vi "niWLAN - 80211abgnIQMeasurementsSettings_5663.vi"(0 "niwlan analysis session":T6, 1 "WLAN Measurement Settings":T1={"OFDM Advanced Controls(11ag)"={"OFDM Auto Compute Acquisition Length Enabled"=0, "OFDM Maximum Symbols Used"=0, "OFDM Time Tracking Enabled"=0, "OFDM Channel Tracking Enabled"=0, "OFDM Amplitude Tracking Enabled"=1, "OFDM CFO Estimation Method"=0, "OFDM Phase Tracking Method"=0, "OFDM Header Detection Enabled"=0, "OFDM MAC FCS Check Enabled"=0, "#Avg"=10, "#Iterations"=10}, "DSSS Demod Parameters"={"DSSS Auto Compute Acquisition Length Enabled"=0, "DSSS Equalization Enabled"=0, "DSSS Header Detection Enabled"=0, "DSSS MAC FCS Check Enabled"=0, "DSSS Measurement Start Location"=0, "DSSS Phase Tracking Method"=0, "DSSS Maximum Chips Used"=0, "DSSS Reference Pulse Shaping Filter"=0, "DSSS Reference Pulse Shaping Filter Coefficient"=0.0, "# Avg"=1024, "# Iterations"=1024, "DSSS Power Ramp Enabled"=0}, "OFDM Advanced Controls (11n)"={"OFDM Auto Compute Acquisition Length Enabled"=0, "OFDM Maximum Symbols Used"=0, "OFDM Time Tracking Enabled"=0, "OFDM Channel Tracking Enabled"=0, "OFDM Amplitude Tracking Enabled"=1, "OFDM CFO Estimation Method"=0, "OFDM Phase Tracking Method"=0, "OFDM Header Detection Enabled"=0, "OFDM MAC FCS Check Enabled"=0, "#Avg"=10, "#Iterations"=10}, "OFDM Advanced Controls(11ac)"={"OFDM Auto Compute Acquisition Length Enabled"=0, "OFDM Maximum Symbols Used"=0, "OFDM Time Tracking Enabled"=1, "OFDM Channel Tracking Enabled"=0, "OFDM Amplitude Tracking Enabled"=0, "OFDM CFO Estimation Method"=0, "OFDM Phase Tracking Method"=0, "OFDM Header Detection Enabled"=0, "OFDM MAC FCS Check Enabled"=0, "#Avg"=10, "#Iterations"=10}} {"OFDM Advanced Controls(11ac)"."OFDM Phase Tracking Method" items=["Standard", "Instantaneous", "None", "Standard with Cubic Spline Fit"]; "OFDM Advanced Controls(11ac)"."OFDM CFO Estimation Method" items=["Preamble Only", "Preamble and Data"]; "OFDM Advanced Controls(11ac)"."OFDM Channel Tracking Enabled" items=["False", "True"]; "OFDM Advanced Controls(11ac)"."OFDM Amplitude Tracking Enabled" items=["False", "True"]; "OFDM Advanced Controls(11ac)"."OFDM Time Tracking Enabled" items=["True"=1, "False"=0]; "OFDM Advanced Controls(11ac)"."OFDM Auto Compute Acquisition Length Enabled" items=["False", "True"]; "OFDM Advanced Controls(11ac)"."OFDM MAC FCS Check Enabled" items=["False", "True"]; "OFDM Advanced Controls(11ac)"."OFDM Header Detection Enabled" items=["False", "True"]; "OFDM Advanced Controls (11n)"."OFDM Phase Tracking Method" items=["Standard", "Instantaneous", "None", "Standard with Cubic Spline Fit"]; "OFDM Advanced Controls (11n)"."OFDM CFO Estimation Method" items=["Preamble Only", "Preamble and Data"]; "OFDM Advanced Controls (11n)"."OFDM Channel Tracking Enabled" items=["False", "True"]; "OFDM Advanced Controls (11n)"."OFDM Amplitude Tracking Enabled" items=["False", "True"]; "OFDM Advanced Controls (11n)"."OFDM Time Tracking Enabled" items=["True"=1, "False"=0]; "OFDM Advanced Controls (11n)"."OFDM Auto Compute Acquisition Length Enabled" items=["False", "True"]; "OFDM Advanced Controls (11n)"."OFDM MAC FCS Check Enabled" items=["False", "True"]; "OFDM Advanced Controls (11n)"."OFDM Header Detection Enabled" items=["False", "True"]; "DSSS Demod Parameters"."DSSS Power Ramp Enabled" items=["False", "True"]; "DSSS Demod Parameters"."DSSS Auto Compute Acquisition Length Enabled" items=["False", "True"]; "DSSS Demod Parameters"."DSSS Phase Tracking Method" items=["Standard", "Instantaneous"]; "DSSS Demod Parameters"."DSSS Equalization Enabled" items=["False", "True"]; "DSSS Demod Parameters"."DSSS Reference Pulse Shaping Filter" items=["Rectangular", "Raised Cosine", "Root Raised Cosine", "Gaussian"]; "DSSS Demod Parameters"."DSSS MAC FCS Check Enabled" items=["False", "True"]; "DSSS Demod Parameters"."DSSS Header Detection Enabled" items=["False", "True"]; "OFDM Advanced Controls(11ag)"."OFDM Phase Tracking Method" items=["Standard", "Instantaneous", "None", "Standard with Cubic Spline Fit"]; "OFDM Advanced Controls(11ag)"."OFDM CFO Estimation Method" items=["Preamble Only", "Preamble and Data"]; "OFDM Advanced Controls(11ag)"."OFDM Channel Tracking Enabled" items=["False", "True"]; "OFDM Advanced Controls(11ag)"."OFDM Amplitude Tracking Enabled" items=["False", "True"]; "OFDM Advanced Controls(11ag)"."OFDM Time Tracking Enabled" items=["True"=1, "False"=0]; "OFDM Advanced Controls(11ag)"."OFDM Auto Compute Acquisition Length Enabled" items=["False", "True"]; "OFDM Advanced Controls(11ag)"."OFDM MAC FCS Check Enabled" items=["False", "True"]; "OFDM Advanced Controls(11ag)"."OFDM Header Detection Enabled" items=["False", "True"]}, 2 "Measurement Type":T4(ring), 5 "TV Parameters(DataType)":T5 {"Standard" items=["80211A/G/J/P OFDM", "80211B/G DSSS", "80211G DSSSOFDM", "80211N MIMOOFDM", "80211AC MIMOOFDM"]; "OFDM Data Rate (Mbps)" items=["6", "9", "12", "18", "24", "36", "48", "54"]; "80211n PLCP Frame Format" items=["Mixed Format", "Greenfield Format"]; "FEC Coding Type" items=["BCC", "LDPC"]; "DSSS Data Rate (Mbps)" items=["1", "2", "5.5 CCK", "5.5 PBCC", "11 CCK", "11 PBCC", "22", "33"]}, 7 "Set TV ?":bool, 11 "error in":errorcluster, 13 "Cal Routine ?":bool) -> (4 "niWLAN session":T6, 15 "error out":errorcluster)   [LabVIEW 2011]
uses:
  <vilib>/RF Toolkits/WLAN/analysis/controls/wlanv1 Analysis Refnum.ctl
  TV/RW/Includes/WLAN - TV - RW - INC - TV_DataType_Cluster.ctl
  TV/RW/Includes/WLAN - TV - RW - INC - Tx_Measurement_Cluster.ctl
  TV/RW/Includes/WLAN - TV - RW - INC - TV_OFDM Demod.ctl
  TV/RW/Includes/WLAN - TV - RW - INC - TV_DSSS Demod.ctl
  Program Files/National Instruments/LabVIEW 2011/resource/objmgr/niWLANAnalysis.rc
panel:
  out "Standard":i32(ring) items=["80211A/G/J/P OFDM", "80211B/G DSSS", "80211G DSSSOFDM", "80211N MIMOOFDM", "80211AC MIMOOFDM"]
  # "Hardware Configuration"
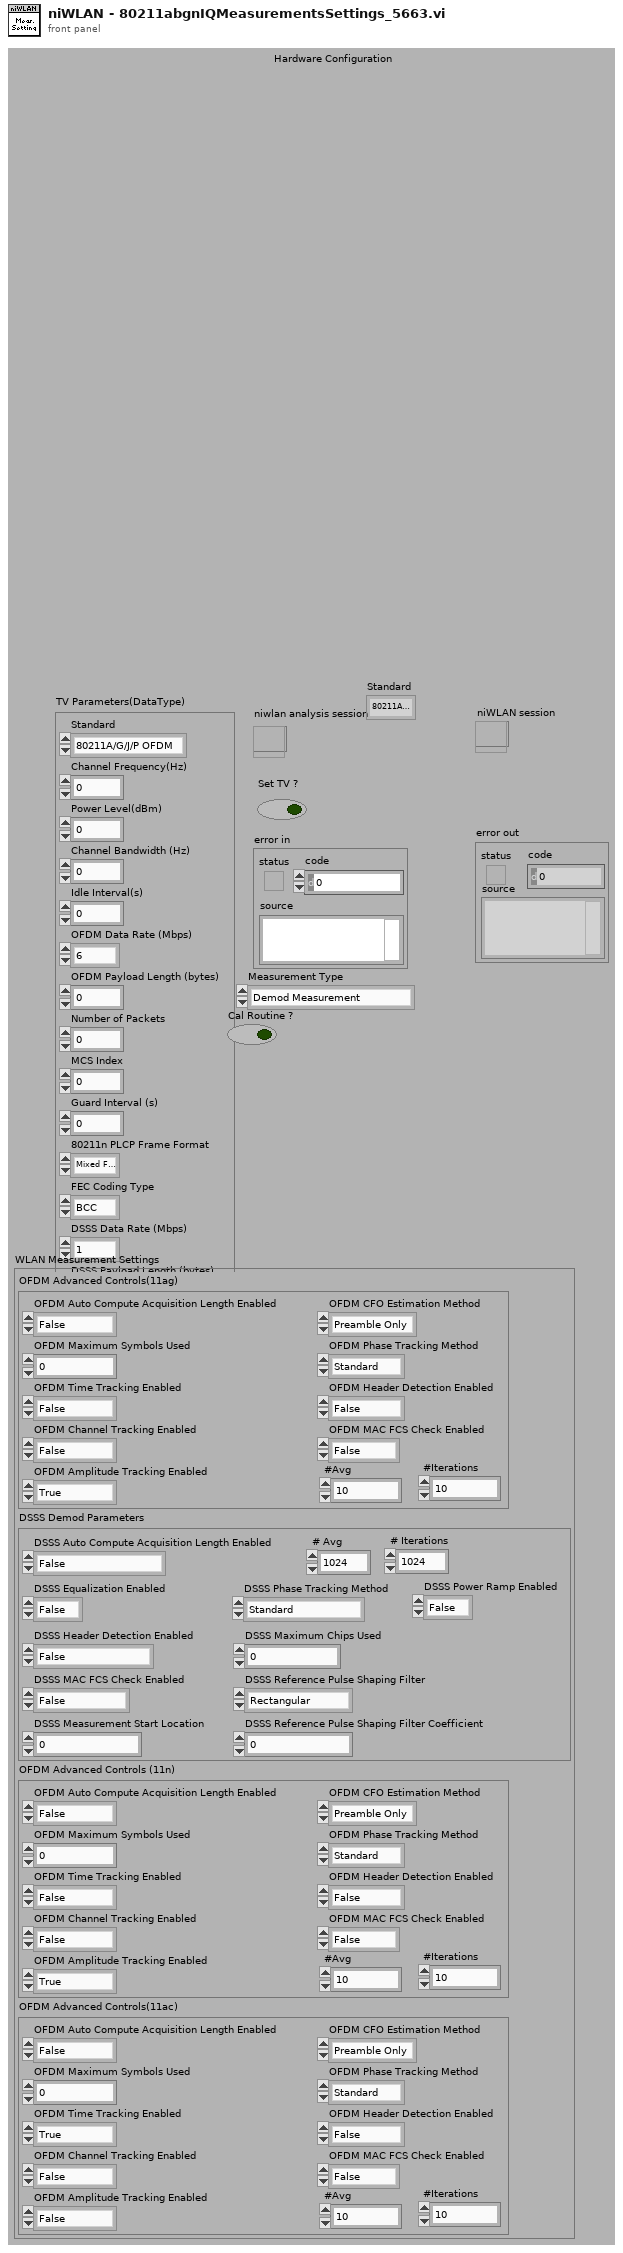
[diagram p1: front panel]
types:
  T1 = typedef "WLAN - TV - RW - INC - Tx_Measurement_Cluster.ctl" = cluster{"OFDM Advanced Controls(11ag)":T2, "DSSS Demod Parameters":T3, "OFDM Advanced Controls (11n)":T2, "OFDM Advanced Controls(11ac)":cluster{"OFDM Auto Compute Acquisition Length Enabled":i32, "OFDM Maximum Symbols Used":i32, "OFDM Time Tracking Enabled":i32, "OFDM Channel Tracking Enabled":i32, "OFDM Amplitude Tracking Enabled":i32, "OFDM CFO Estimation Method":i32, "OFDM Phase Tracking Method":i32, "OFDM Header Detection Enabled":i32, "OFDM MAC FCS Check Enabled":i32, "#Avg":i32, "#Iterations":i32}}
  T2 = typedef "WLAN - TV - RW - INC - TV_OFDM Demod.ctl" = cluster{"OFDM Auto Compute Acquisition Length Enabled":i32, "OFDM Maximum Symbols Used":i32, "OFDM Time Tracking Enabled":i32, "OFDM Channel Tracking Enabled":i32, "OFDM Amplitude Tracking Enabled":i32, "OFDM CFO Estimation Method":i32, "OFDM Phase Tracking Method":i32, "OFDM Header Detection Enabled":i32, "OFDM MAC FCS Check Enabled":i32, "#Avg":i32, "#Iterations":i32}
  T3 = typedef "WLAN - TV - RW - INC - TV_DSSS Demod.ctl" = cluster{"DSSS Auto Compute Acquisition Length Enabled":i32, "DSSS Equalization Enabled":i32, "DSSS Header Detection Enabled":i32, "DSSS MAC FCS Check Enabled":i32, "DSSS Measurement Start Location":i32, "DSSS Phase Tracking Method":i32, "DSSS Maximum Chips Used":i32, "DSSS Reference Pulse Shaping Filter":i32, "DSSS Reference Pulse Shaping Filter Coefficient":dbl, "# Avg":i32, "# Iterations":i32, "DSSS Power Ramp Enabled":i32}
  T4 = enum16{"Demod Measurement", "Spectrum Measurement"}
  T5 = typedef "WLAN - TV - RW - INC - TV_DataType_Cluster.ctl" = cluster{"Standard":i32, "Channel Frequency(Hz)":dbl, "Power Level(dBm)":dbl, "Channel Bandwidth (Hz)":dbl, "Idle Interval(s)":dbl, "OFDM Data Rate (Mbps)":i32, "OFDM Payload Length (bytes)":i32, "Number of Packets":i32, "MCS Index":i32, "Guard Interval (s)":dbl, "80211n PLCP Frame Format":i32, "FEC Coding Type":i32, "DSSS Data Rate (Mbps)":i32, "DSSS Payload Length (bytes)":i32, "N_SS":i32}
  T6 = typedef "wlanv1 Analysis Refnum.ctl" = refnum<k20>
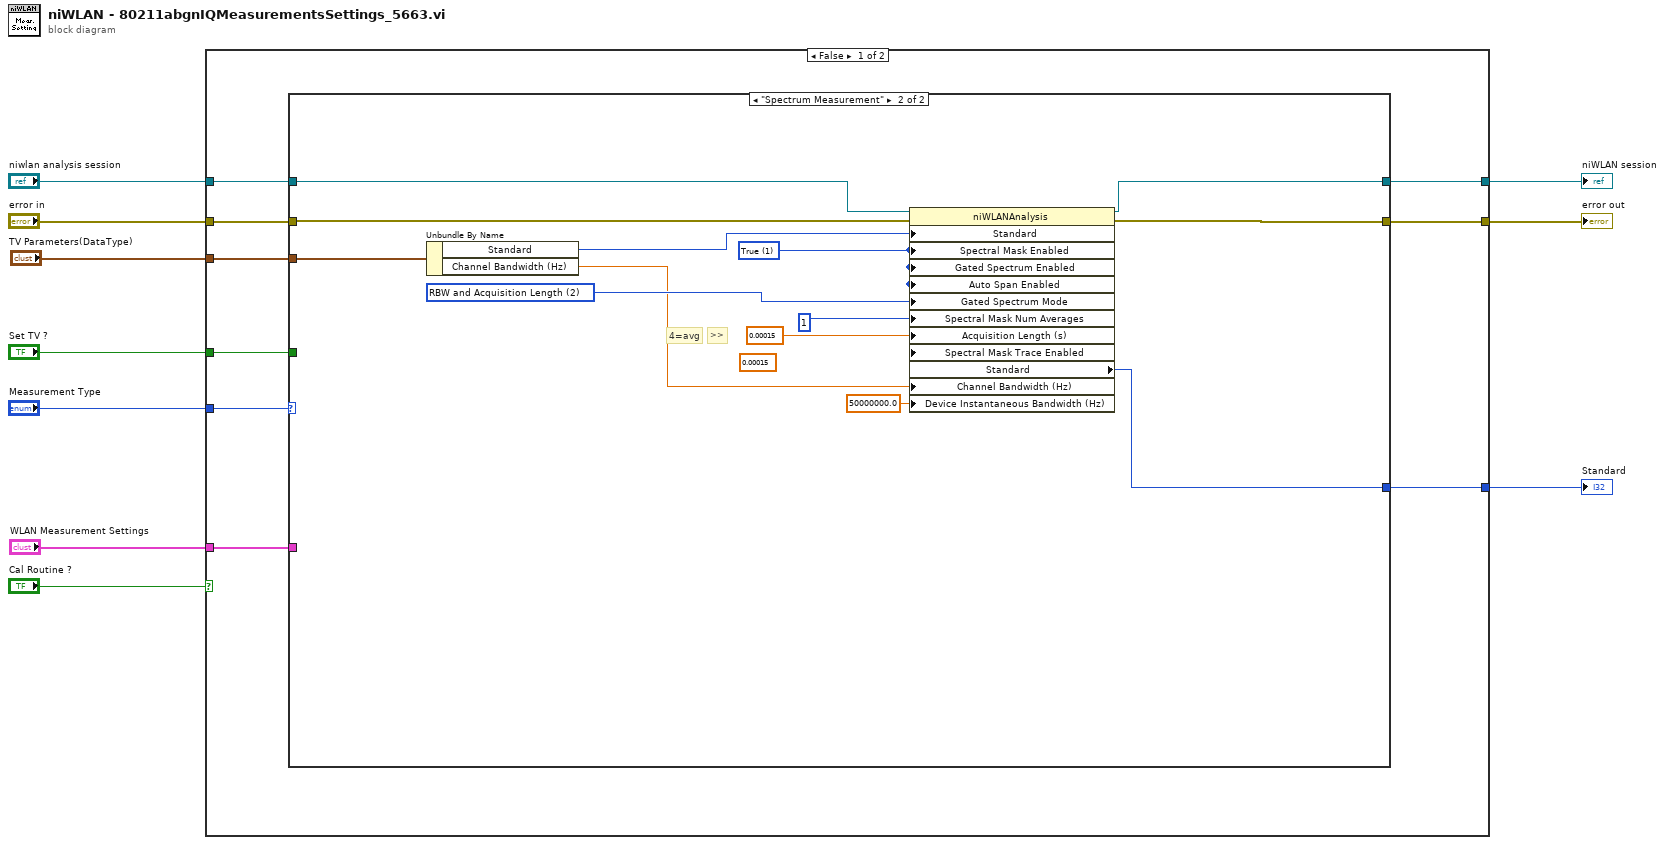
[diagram p0: block diagram]
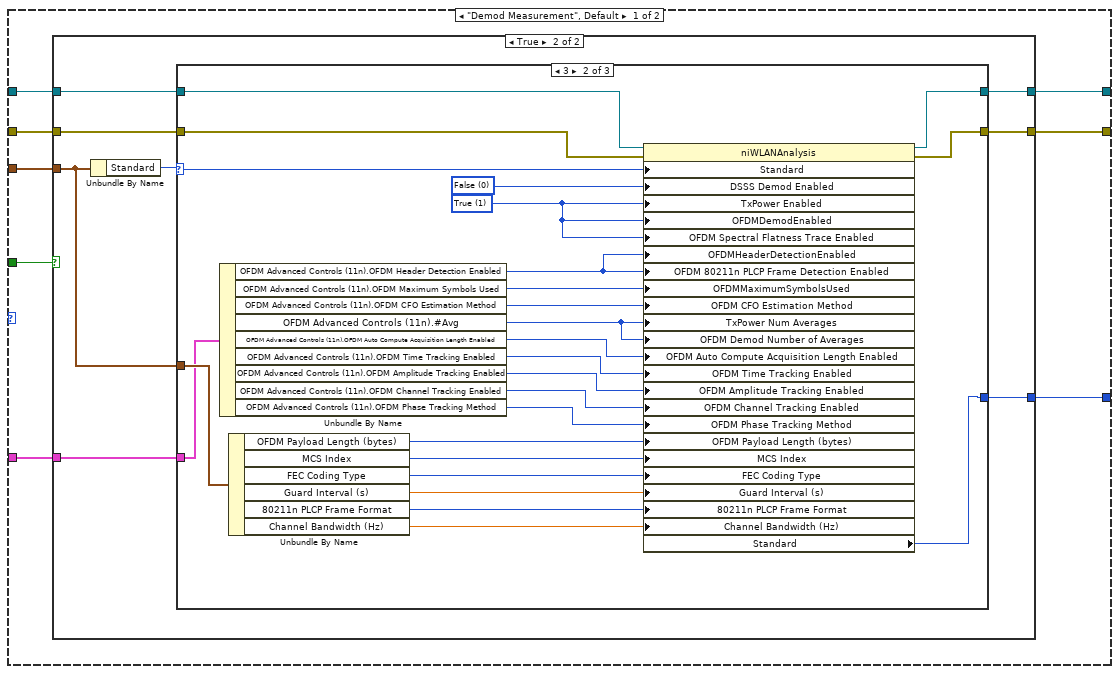
[diagram p2: hidden frame]
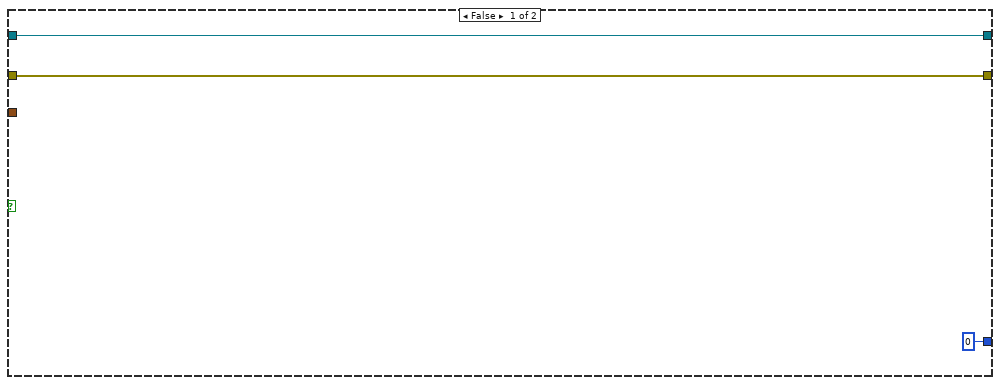
[diagram p3: hidden frame]
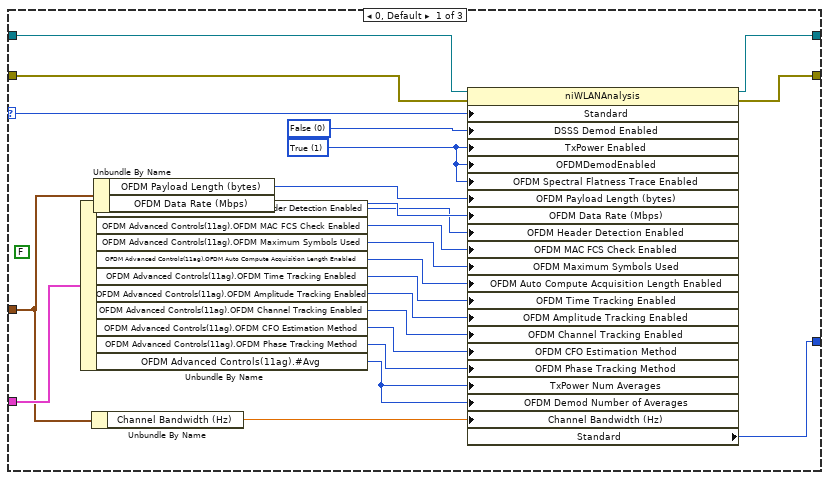
[diagram p4: hidden frame]
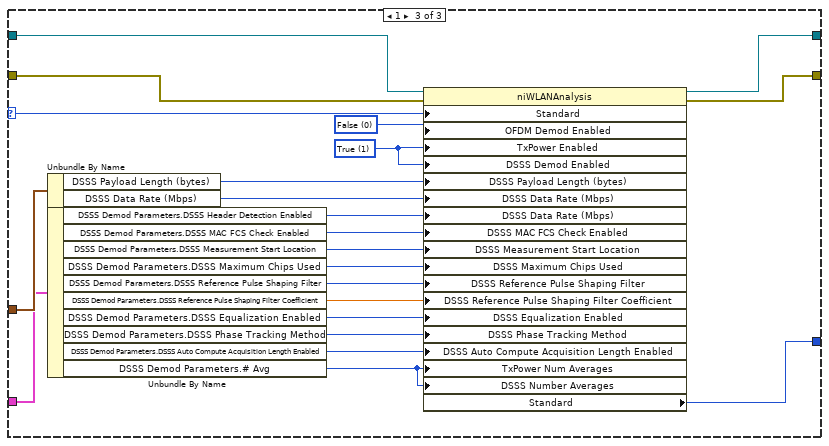
[diagram p5: hidden frame]
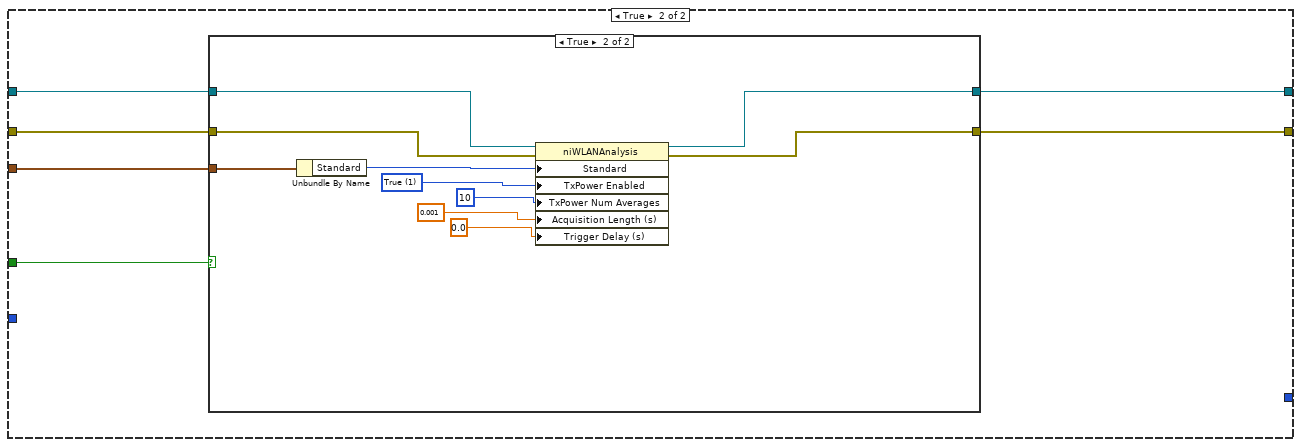
[diagram p6: hidden frame]
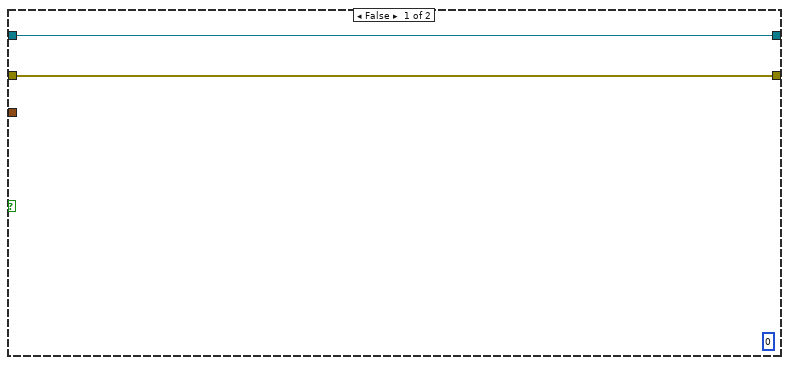
[diagram p7: hidden frame]
diagram:
  n1 = case shown="False" "Cal Routine ?" {
    tunnel: "niwlan analysis session" -> [w19 w127]
    tunnel: "error in" -> [w18 w126]
    tunnel: [w17 w125] -> w8
    tunnel: [w16 w124] -> w7
    tunnel: "TV Parameters(DataType)" -> [w15 w123]
    tunnel: "Set TV ?" -> [w14 w122]
    tunnel: "Measurement Type" -> [w13 _]
    tunnel: [w12 _] -> w3
    tunnel: "WLAN Measurement Settings" -> [w11 _]
    frame False {
      n2 = case shown="\"Spectrum Measurement\"" w13 {
        tunnel: w19 -> [w27 w121]
        tunnel: w18 -> [w26 w120]
        tunnel: [w25 w118] -> w17
        tunnel: [w24 w117] -> w16
        tunnel: w15 -> [w23 w119]
        tunnel: w14 -> [w22 _]
        tunnel: [w21 w116] -> w12
        tunnel: w11 -> [w20 _]
        frame "Demod Measurement", Default {
          n3 = case shown="True" w22 {
            tunnel: w27 -> [w30 w38]
            tunnel: w26 -> [w29 w37]
            tunnel: [w30 w36] -> w25
            tunnel: [w29 w35] -> w24
            tunnel: w23 -> [_ w33]
            tunnel: [0 ("Standard") w32] -> w21
            tunnel: w20 -> [_ w31]
            frame False {
            }
            frame True {
              n4 = Unbundle By Name(w33) -> ("Standard"=w34:i32)
              n5 = case shown="3" w34 {
                selector: w34 -> [w57 w82 w104]
                tunnel: w38 -> [w61 w86 w108]
                tunnel: w37 -> [w60 w85 w107]
                tunnel: [w59 w84 w106] -> w36
                tunnel: [w58 w83 w105] -> w35
                tunnel: w33 -> [w55 w81 w103]
                tunnel: [w54 w74 w87] -> w32
                tunnel: w31 -> [w56 w72 w98]
                frame 0, Default {
                  w51 = 0 items=["False", "True"] ("DSSS Demod Enabled")
                  w50 = 1 items=["False", "True"] ("OFDMDemodEnabled")
                  (unwired) FALSE
                  n6 = Unbundle By Name(w56) -> ("OFDM Advanced Controls(11ag).OFDM Header Detection Enabled"=w49:i32, "OFDM Advanced Controls(11ag).OFDM MAC FCS Check Enabled"=w48:i32, "OFDM Advanced Controls(11ag).OFDM Maximum Symbols Used"=w47:i32, "OFDM Advanced Controls(11ag).OFDM Auto Compute Acquisition Length Enabled"=w39:i32, "OFDM Advanced Controls(11ag).OFDM Time Tracking Enabled"=w46:i32, "OFDM Advanced Controls(11ag).OFDM Amplitude Tracking Enabled"=w45:i32, "OFDM Advanced Controls(11ag).OFDM Channel Tracking Enabled"=w44:i32, "OFDM Advanced Controls(11ag).OFDM CFO Estimation Method"=w43:i32, "OFDM Advanced Controls(11ag).OFDM Phase Tracking Method"=w42:i32, "OFDM Advanced Controls(11ag).#Avg"=w41:i32)
                  n7 = Unbundle By Name(w55) -> ("Channel Bandwidth (Hz)"=w40:dbl)
                  n8 = Unbundle By Name(w55) -> ("OFDM Payload Length (bytes)"=w53:i32, "OFDM Data Rate (Mbps)"=w52:i32)
                  n9 = property class="niWLANAnalysis"(reference=w61, error in=w60, "Standard"=w57, "DSSS Demod Enabled"=w51, "TxPower Enabled"=w50, "OFDMDemodEnabled"=w50, "OFDM Spectral Flatness Trace Enabled"=w50, "OFDM Payload Length (bytes)"=w53, "OFDM Data Rate (Mbps)"=w52, "OFDM Header Detection Enabled"=w49, "OFDM MAC FCS Check Enabled"=w48, "OFDM Maximum Symbols Used"=w47, "OFDM Auto Compute Acquisition Length Enabled"=w39, "OFDM Time Tracking Enabled"=w46, "OFDM Amplitude Tracking Enabled"=w45, "OFDM Channel Tracking Enabled"=w44, "OFDM CFO Estimation Method"=w43, "OFDM Phase Tracking Method"=w42, "TxPower Num Averages"=w41, "OFDM Demod Number of Averages"=w41, "Channel Bandwidth (Hz)"=w40) -> (reference out=w59:T6, error out=w58:errorcluster, "Standard"=w54:i32)
                }
                frame 3 {
                  w73 = 0 items=["False", "True"] ("OFDMDemodEnabled")
                  w62 = 1 items=["False", "True"] ("OFDMDemodEnabled")
                  n10 = Unbundle By Name(w72) -> ("OFDM Advanced Controls (11n).OFDM Header Detection Enabled"=w63:i32, "OFDM Advanced Controls (11n).OFDM Maximum Symbols Used"=w71:i32, "OFDM Advanced Controls (11n).OFDM CFO Estimation Method"=w70:i32, "OFDM Advanced Controls (11n).#Avg"=w69:i32, "OFDM Advanced Controls (11n).OFDM Auto Compute Acquisition Length Enabled"=w68:i32, "OFDM Advanced Controls (11n).OFDM Time Tracking Enabled"=w67:i32, "OFDM Advanced Controls (11n).OFDM Amplitude Tracking Enabled"=w66:i32, "OFDM Advanced Controls (11n).OFDM Channel Tracking Enabled"=w65:i32, "OFDM Advanced Controls (11n).OFDM Phase Tracking Method"=w64:i32)
                  n11 = Unbundle By Name(w81) -> ("OFDM Payload Length (bytes)"=w80:i32, "MCS Index"=w79:i32, "FEC Coding Type"=w78:i32, "Guard Interval (s)"=w77:dbl, "80211n PLCP Frame Format"=w76:i32, "Channel Bandwidth (Hz)"=w75:dbl)
                  n12 = property class="niWLANAnalysis"(reference=w86, error in=w85, "Standard"=w82, "DSSS Demod Enabled"=w73, "TxPower Enabled"=w62, "OFDMDemodEnabled"=w62, "OFDM Spectral Flatness Trace Enabled"=w62, "OFDMHeaderDetectionEnabled"=w63, "OFDM 80211n PLCP Frame Detection Enabled"=w63, "OFDMMaximumSymbolsUsed"=w71, "OFDM CFO Estimation Method"=w70, "TxPower Num Averages"=w69, "OFDM Demod Number of Averages"=w69, "OFDM Auto Compute Acquisition Length Enabled"=w68, "OFDM Time Tracking Enabled"=w67, "OFDM Amplitude Tracking Enabled"=w66, "OFDM Channel Tracking Enabled"=w65, "OFDM Phase Tracking Method"=w64, "OFDM Payload Length (bytes)"=w80, "MCS Index"=w79, "FEC Coding Type"=w78, "Guard Interval (s)"=w77, "80211n PLCP Frame Format"=w76, "Channel Bandwidth (Hz)"=w75) -> (reference out=w84:T6, error out=w83:errorcluster, "Standard"=w74:i32)
                }
                frame 1 {
                  w99 = 0 items=["False", "True"] ("OFDM Demod Enabled")
                  w100 = 1 items=["False", "True"] ("OFDMDemodEnabled")
                  n13 = Unbundle By Name(w103) -> ("DSSS Payload Length (bytes)"=w102:i32, "DSSS Data Rate (Mbps)"=w101:i32)
                  n14 = Unbundle By Name(w98) -> ("DSSS Demod Parameters.DSSS Header Detection Enabled"=w95:i32, "DSSS Demod Parameters.DSSS MAC FCS Check Enabled"=w94:i32, "DSSS Demod Parameters.DSSS Measurement Start Location"=w93:i32, "DSSS Demod Parameters.DSSS Maximum Chips Used"=w92:i32, "DSSS Demod Parameters.DSSS Reference Pulse Shaping Filter"=w96:i32, "DSSS Demod Parameters.DSSS Reference Pulse Shaping Filter Coefficient"=w97:dbl, "DSSS Demod Parameters.DSSS Equalization Enabled"=w91:i32, "DSSS Demod Parameters.DSSS Phase Tracking Method"=w90:i32, "DSSS Demod Parameters.DSSS Auto Compute Acquisition Length Enabled"=w89:i32, "DSSS Demod Parameters.# Avg"=w88:i32)
                  n15 = property class="niWLANAnalysis"(reference=w108, error in=w107, "Standard"=w104, "OFDM Demod Enabled"=w99, "TxPower Enabled"=w100, "DSSS Demod Enabled"=w100, "DSSS Payload Length (bytes)"=w102, "DSSS Data Rate (Mbps)"=w101, "DSSS Data Rate (Mbps)"=w95, "DSSS MAC FCS Check Enabled"=w94, "DSSS Measurement Start Location"=w93, "DSSS Maximum Chips Used"=w92, "DSSS Reference Pulse Shaping Filter"=w96, "DSSS Reference Pulse Shaping Filter Coefficient"=w97, "DSSS Equalization Enabled"=w91, "DSSS Phase Tracking Method"=w90, "DSSS Auto Compute Acquisition Length Enabled"=w89, "TxPower Num Averages"=w88, "DSSS Number Averages"=w88) -> (reference out=w106:T6, error out=w105:errorcluster, "Standard"=w87:i32)
                }
              }
            }
          }
        }
        frame "Spectrum Measurement" {
          (unwired) 0.00015 ("Acquisition Length (s)")
          w113 = 2 items=["RBW", "Acquisition Length", "RBW and Acquisition Length"] ("Gated Spectrum Mode")
          w111 = 1 items=["False", "True"] ("OFDMDemodEnabled")
          # "4=avg"
          # ">>"
          n16 = Unbundle By Name(w119) -> ("Standard"=w115:i32, "Channel Bandwidth (Hz)"=w110:dbl)
          n17 = property class="niWLANAnalysis"(reference=w121, error in=w120, "Standard"=w115, "Spectral Mask Enabled"=w111, "Gated Spectrum Enabled"=w111, "Auto Span Enabled"=w111, "Gated Spectrum Mode"=w113, "Spectral Mask Num Averages"=1 ("Averages"), "Acquisition Length (s)"=0.00015, "Spectral Mask Trace Enabled"=w111, "Channel Bandwidth (Hz)"=w110, "Device Instantaneous Bandwidth (Hz)"=50000000.0) -> (reference out=w118:T6, error out=w117:errorcluster, "Standard"=w116:i32)
        }
      }
    }
    frame True {
      n18 = case shown="True" w122 {
        tunnel: w127 -> [w129 w139]
        tunnel: w126 -> [w128 w138]
        tunnel: [w129 w137] -> w125
        tunnel: [w128 w136] -> w124
        tunnel: w123 -> [_ w134]
        frame False {
          (unwired) 0 ("Standard")
        }
        frame True {
          w131 = 1 items=["False", "True"] ("OFDMDemodEnabled")
          n19 = Unbundle By Name(w134) -> ("Standard"=w135:i32)
          n20 = property class="niWLANAnalysis"(reference=w139, error in=w138, "Standard"=w135, "TxPower Enabled"=w131, "TxPower Num Averages"=10, "Acquisition Length (s)"=0.001, "Trigger Delay (s)"=0.0 ("Trigger Delay (sec)")) -> (reference out=w137:T6, error out=w136:errorcluster)
        }
      }
    }
  }
  "error out" <- w7
  "niWLAN session" <- w8
  "Standard" <- w3
